vi "RPC__method Register.vi"(8 "error in (no error)":errorcluster, 11 "OOP Server in":refnum<class "OOP Server.lvclass">) -> (0 "error out":errorcluster, 3 "OOP Server out":refnum<class "OOP Server.lvclass">)   [LabVIEW 2019, in "OOP Server.lvclass"]
uses:
  OOP Server.lvclass
  gRPC interface/Server API/typeDefs/grpcId.ctl
  OOP Server.lvclass/OOP Server.ctl
  RPC Messages/ServerEvent/ServerEvent_Data.ctl
  gRPC interface/gprc-lvsupport.lvlib
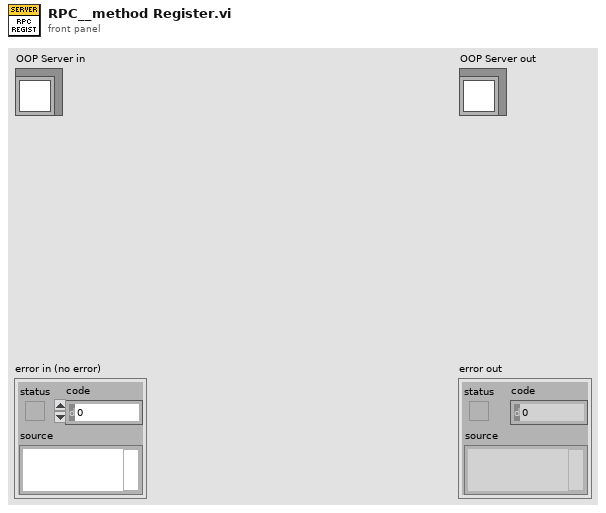
[diagram p1: front panel]
types:
  T1 = typedef "gprc-lvsupport.lvlib/grpcId.ctl" = u64
  T2 = typedef "OOP Server.lvclass/ServerEvent_Data.ctl" = cluster{"eventData":string, "serverId":i32, "status":i32}
  T3 = typedef "OOP Server.lvclass/Server Internal UEs.ctl" = cluster{"Invoke Internal UE":refnum<user-event>, "Query Internal UE":refnum<user-event>, "Register Internal UE":refnum<user-event>}
  T4 = typedef "OOP Server.lvclass/Server gRPC UEs.ctl" = cluster{"Invoke gRPC UEs":T5, "Query gRPC UEs":T5, "Register gRPC UEs":T5}
  T5 = typedef "gprc-lvsupport.lvlib/gRPCId Cluster UE.ctl" = refnum<user-event>
  T6 = typedef "OOP Server.lvclass/RegistrationRequest_Data.ctl" = cluster{"eventName":string}
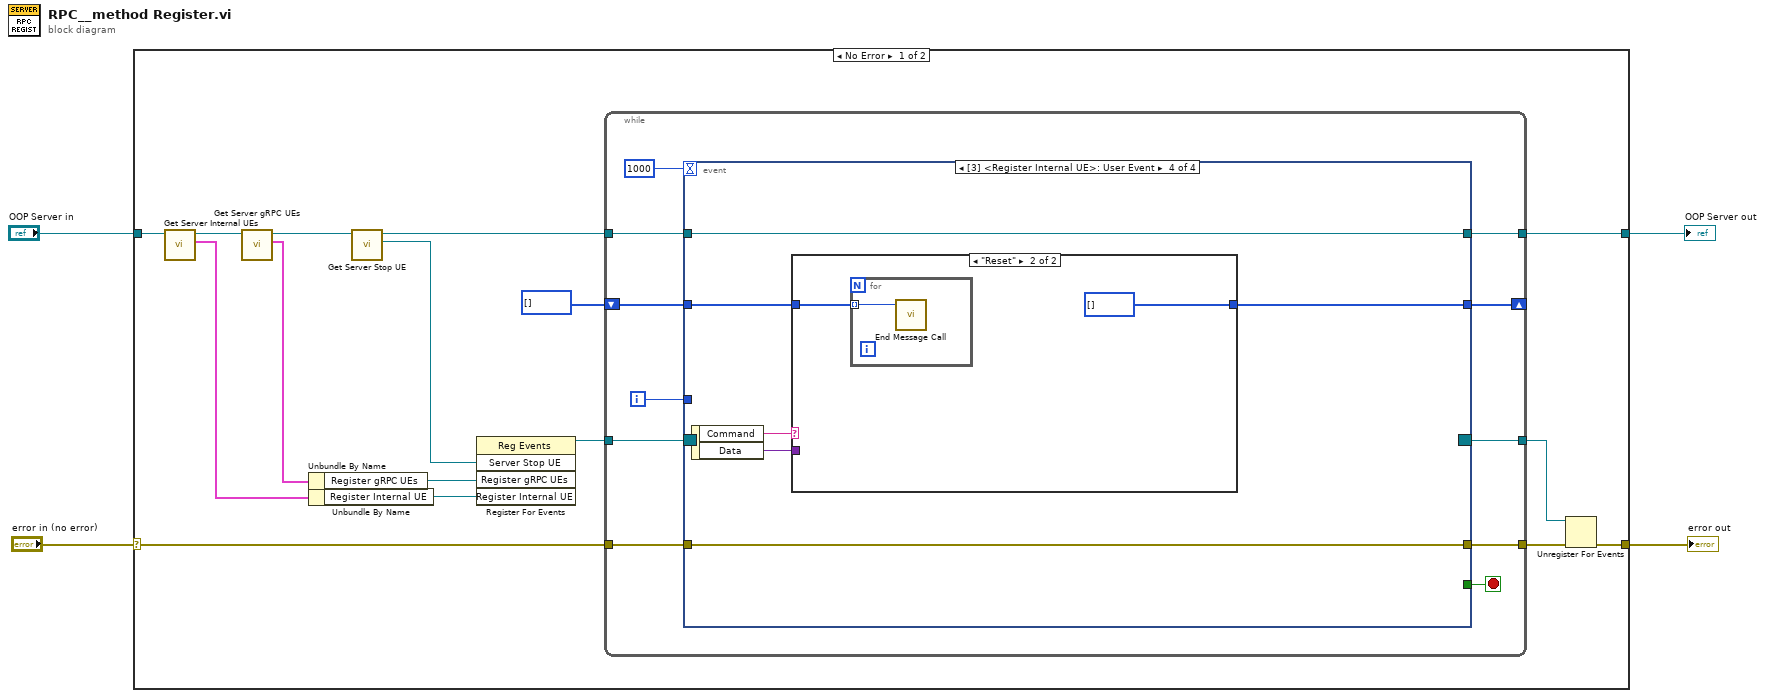
[diagram p0: block diagram]
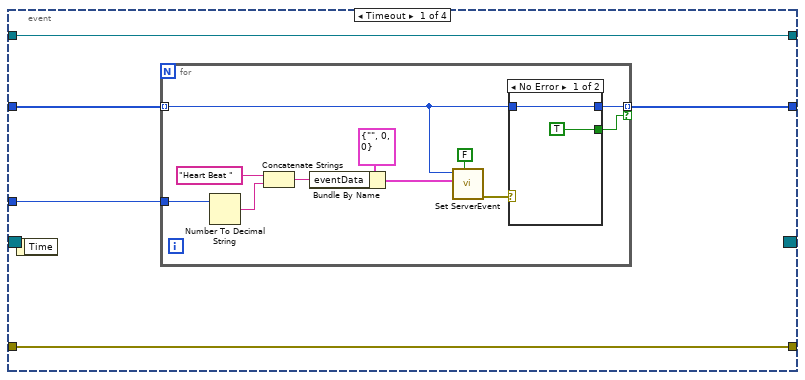
[diagram p2: hidden frame]
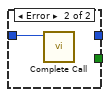
[diagram p3: hidden frame]
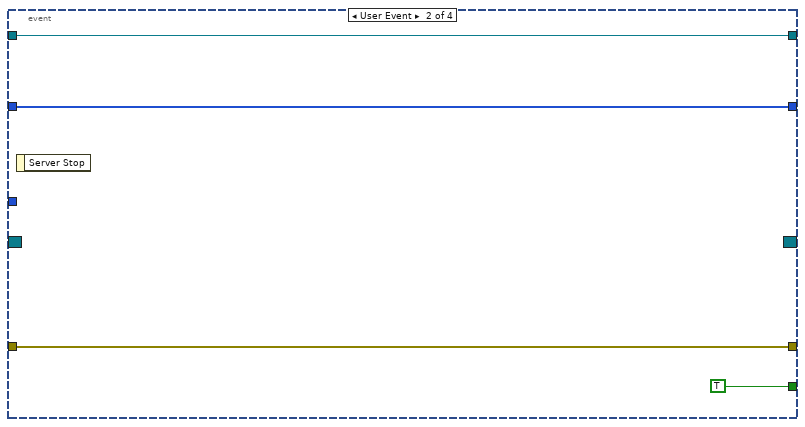
[diagram p4: hidden frame]
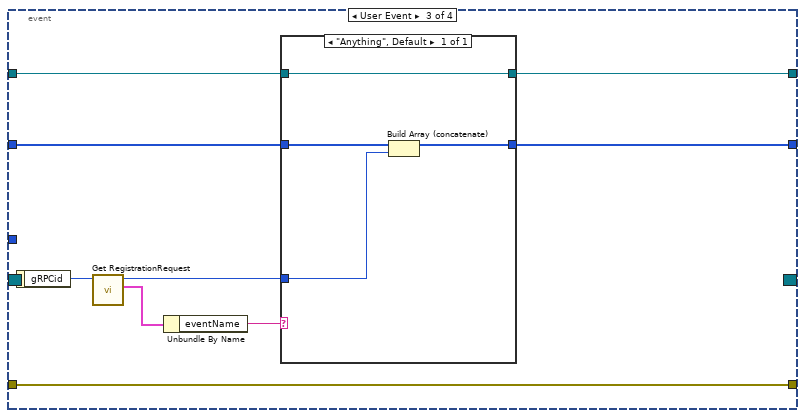
[diagram p5: hidden frame]
diagram:
  n1 = case shown="No Error" "error in (no error)" {
    selector: "error in (no error)" -> [w11 w79]
    tunnel: [w9 w79] -> w3
    tunnel: [w6 w78] -> w1
    tunnel: "OOP Server in" -> [w15 w78]
    frame No Error {
      n2 = call "Get Server Internal UEs.vi"("OOP Server in"=w15) -> ("Server Internal UEs"=w13:T3, "OOP Server out"=w14:refnum<class "OOP Server.lvclass">)  [unwired: 9 in]
      n3 = call "Get Server gRPC UEs.vi"("OOP Server in"=w14) -> ("Server gRPC UEs"=w17:T4, "OOP Server out"=w20:refnum<class "OOP Server.lvclass">)  [unwired: 9 in]
      n4 = Unbundle By Name(w17) -> ("Register gRPC UEs"=w16:T5)
      n5 = Unbundle By Name(w13) -> ("Register Internal UE"=w12:refnum<user-event>)
      n6 = call "Get Server Stop UE.vi"("OOP Server in"=w20) -> ("Server Stop UE"=w19:refnum<user-event>, "OOP Server out"=w7:refnum<class "OOP Server.lvclass">)  [unwired: 9 in]
      n7 = register-events(w19, w16, w12) -> (reference out=w18:refnum<event-registration>)  [unwired: 2 in, 1 out]
      n8 = while {
        tunnel: w18 -> [w31]
        tunnel: w11 -> [w29]
        tunnel: [w28] -> w10
        tunnel: [w27] -> w8
        tunnel: w7 -> [w24]
        tunnel: [w23] -> w6
        shift-right: [w21] -> _
        shift-left: T1[] [] -> [w22]
        i -> [w26]
        stop <- w30 stop-if-true
        n9 = event shown="[3] <Register Internal UE>: User Event" {
          selector: w31 -> [_ _ _ _]
          dyn-events: [_ _ _ _] -> w27
          timeout: 1000 -> [_ _ _ _]
          tunnel: [_ TRUE _ _] -> w30
          tunnel: w29 -> [w35 w53 w63 w73]
          tunnel: [w35 w53 w63 w73] -> w28
          tunnel: w26 -> [w36 _ _ _]
          tunnel: w24 -> [w34 w52 w58 w72]
          tunnel: [w34 w52 w57 w72] -> w23
          tunnel: w22 -> [w33 w51 w56 w69]
          tunnel: [w32 w51 w55 w68] -> w21
          event Timeout {
            n10 = event-data() -> ()  [unwired: 1 in, 1 out]
            n11 = for {
              tunnel: [w38] -> w32 mode=indexing if=w40
              tunnel: w36 -> [w42]
              tunnel: w33 -> [w39] mode=indexing
              n12 = Number To Decimal String(number=w42) -> (decimal integer string=w47:string)  [unwired: 1 in]
              n13 = Concatenate Strings("Heart Beat " ("eventdata"), w47) -> (w44:string)
              n14 = Bundle By Name(cluster=T2 {"eventData"="", "serverId"=0, "status"=0} ("ServerEvent_Data"), "eventData"=w44) -> (w43:T2)
              n15 = call "Set ServerEvent.vi"("Complete Call (T)"=FALSE, "ServerEvent_Data"=w43, "gRPCid in"=w39) -> ("error out"=w41:errorcluster)  [unwired: 8 in]
              n16 = case shown="No Error" w41 {
                tunnel: [TRUE _] -> w40
                tunnel: w39 -> [w48 w50]
                tunnel: [w48 _] -> w38
                frame No Error {
                }
                frame Error {
                  n17 = call "Complete Call.vi"("gRPCid"=w50) -> ()  [unwired: 9 in, 1 out]
                }
              }
            }
          }
          event User Event {
            n18 = event-data() -> ()  [unwired: 1 in, 1 out]
          }
          event User Event {
            n19 = event-data() -> ("gRPCid"=w59:T1)  [unwired: 1 in]
            n20 = call "Get RegistrationRequest.vi"("gRPCid in"=w59) -> ("Request Data"=w62:T6, "gRPCid out"=w60:T1)  [unwired: 8 in, 1 out]
            n21 = Unbundle By Name(w62) -> ("eventName"=w61:string)
            n22 = case shown="\"Anything\", Default" w61 {
              tunnel: w60 -> [w66]
              tunnel: w58 -> [w64]
              tunnel: [w64] -> w57
              tunnel: w56 -> [w67]
              tunnel: [w65] -> w55
              frame "Anything", Default {
                n23 = Build Array (concatenate)(w67, w66) -> (w65:T1[])
              }
            }
          }
          event User Event {
            n24 = event-data() -> ("Command"=w71:string, "Data"=w70:variant)  [unwired: 1 in]
            n25 = case shown="\"Reset\"" w71 {
              tunnel: w70 -> [_ _]
              tunnel: w69 -> [w74 w75]
              tunnel: [w74 T1[] []] -> w68
              frame "None", Default {
              }
              frame "Reset" {
                n26 = for {
                  tunnel: w75 -> [w77] mode=indexing
                  n27 = call "End Message Call.vi"("gRPCid"=w77) -> ()  [unwired: 10 in, 1 out]
                }
              }
            }
          }
        }
      }
      n28 = Unregister For Events(event registration refnum=w8, error in=w10) -> (error out=w9:errorcluster)
    }
    frame Error {
    }
  }
  "error out" <- w3
  "OOP Server out" <- w1
